vi "Asana Authentication.vi"(8 "error in (no error)":errorcluster, 9 "Authentication Info":T1={"Client ID"="", "Client Secret"="", "Redirect URI"="", "Token Endpoint"="https://app.asana.com/-/oauth_token", "Scope"=""}, 11 "Asana in":refnum<class "Asana.lvclass">) -> (0 "error out":errorcluster, 2 "Timeout":dbl, 3 "Asana out":refnum<class "Asana.lvclass">)   [LabVIEW 2016, in "Asana.lvclass"]
uses:
  levylab_expt_transport/src/Control Experiment/subVIs/Asana/Asana.lvclass
  OAuth/OO OAuth/scope_needed.ctl
  levylab_expt_transport/src/Control Experiment/subVIs/Asana/Asana.lvclass/Asana.ctl
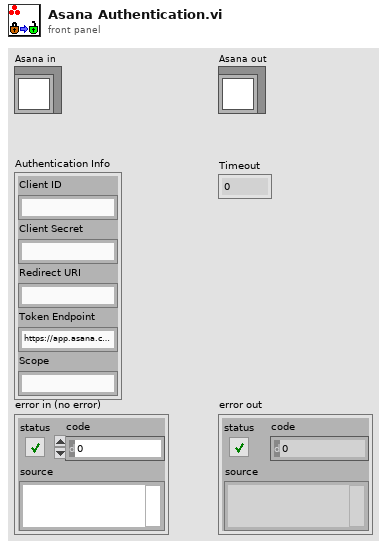
[diagram p1: front panel]
types:
  T1 = cluster{"Client ID":string, "Client Secret":string, "Redirect URI":string, "Token Endpoint":string, "Scope":string}
  T2 = typedef "scope_needed.ctl" = enum16{"No", "Yes"}
  T3 = typedef "REST Client.lvlib/REST Client.lvclass/HTTP Header.ctl" = cluster{"header":string, "value":string}
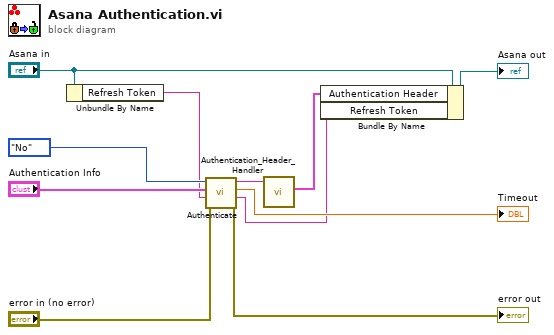
[diagram p0: block diagram]
diagram:
  n1 = Unbundle By Name("Asana in") -> ("Refresh Token"=w4:string)
  n2 = call "Authenticate.vi"("error in (no error)"="error in (no error)", "Refresh Token"=w4, "Authentication Info"="Authentication Info", "Scope Needed?"=scope_needed."No") -> ("error out"=→"error out":errorcluster, "Refresh Token"=w1:string, "Timeout"=→"Timeout":dbl, "Access Token"=w11:string)  [unwired: 4 in]
  n3 = call "Authentication_Header_Handler.vi"("String"=w11) -> ("output array"=w6:T3[])  [unwired: 10 in]
  n4 = Bundle By Name(cluster="Asana in", "Authentication Header"=w6, "Refresh Token"=w1) -> (→"Asana out":refnum<class "Asana.lvclass">)
